vi "ParseL.vi"(1 "String":string="*IDN?\n") -> (6 "Estado":string, 7 "LIM V":string, 11 "LIM A":string, 13 "LIM W":string, 14 "V":string, 15 "A":string, 16 "W":string, 17 "V Control":bool, 18 "A Control":bool, 19 "W Control":bool)   [LabVIEW 2011]
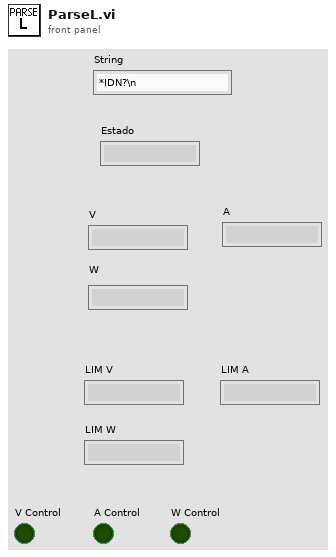
[diagram p1: front panel]
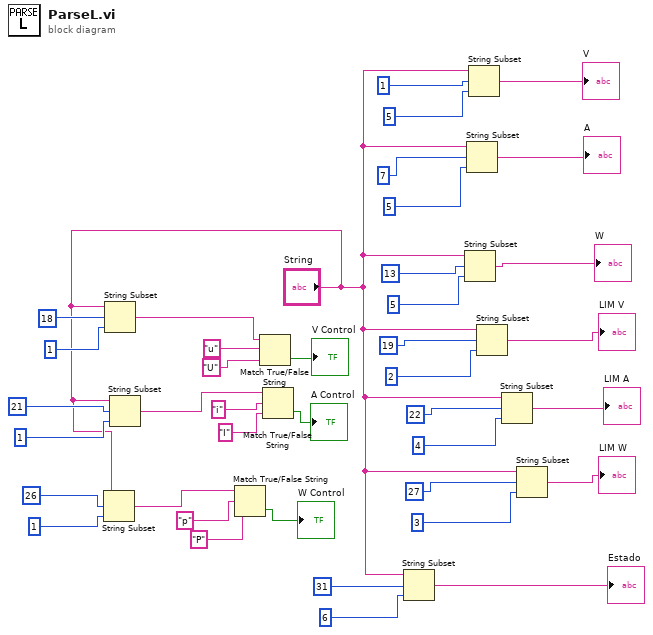
[diagram p0: block diagram]
diagram:
  n1 = String Subset(string="String", offset (0)=26, length (rest)=1) -> (substring=w8:string)
  n2 = String Subset(string="String", offset (0)=18, length (rest)=1) -> (substring=w10:string)
  n3 = String Subset(string="String", offset (0)=21, length (rest)=1) -> (substring=w9:string)
  n4 = Match True/False String(2:"P", 3:"p", 4:w8) -> (0:→"W Control":bool)  [unwired: 1 out]
  n5 = Match True/False String(2:"U", 3:"u", 4:w10) -> (0:→"V Control":bool)  [unwired: 1 out]
  n6 = Match True/False String(2:"I", 3:"i", 4:w9) -> (0:→"A Control":bool)  [unwired: 1 out]
  n7 = String Subset(string="String", offset (0)=31, length (rest)=6) -> (substring=→"Estado":string)
  n8 = String Subset(string="String", offset (0)=13, length (rest)=5) -> (substring=→"W":string)
  n9 = String Subset(string="String", offset (0)=7, length (rest)=5) -> (substring=→"A":string)
  n10 = String Subset(string="String", offset (0)=1, length (rest)=5) -> (substring=→"V":string)
  n11 = String Subset(string="String", offset (0)=19, length (rest)=2) -> (substring=→"LIM V":string)
  n12 = String Subset(string="String", offset (0)=22, length (rest)=4) -> (substring=→"LIM A":string)
  n13 = String Subset(string="String", offset (0)=27, length (rest)=3) -> (substring=→"LIM W":string)
